vi "Log Alarm FGV.vi"(8 "error in (no error)":errorcluster, 9 "Alarm":T1, 10 "Path":path, 11 "Operation":T2) -> (0 "error out":errorcluster)   [LabVIEW 2021, in "Dynamic Shared Variables.lvlib"]
doc: "Creates, writes and closes a CSV file that contains information on alarm transitions (i.e. active, ack, cleared)."
uses:
  Dynamic Shared Variables.lvlib
  Alarm Log Operation Enum.ctl
  Tag VIs/Tag FGV Operation Enum.ctl
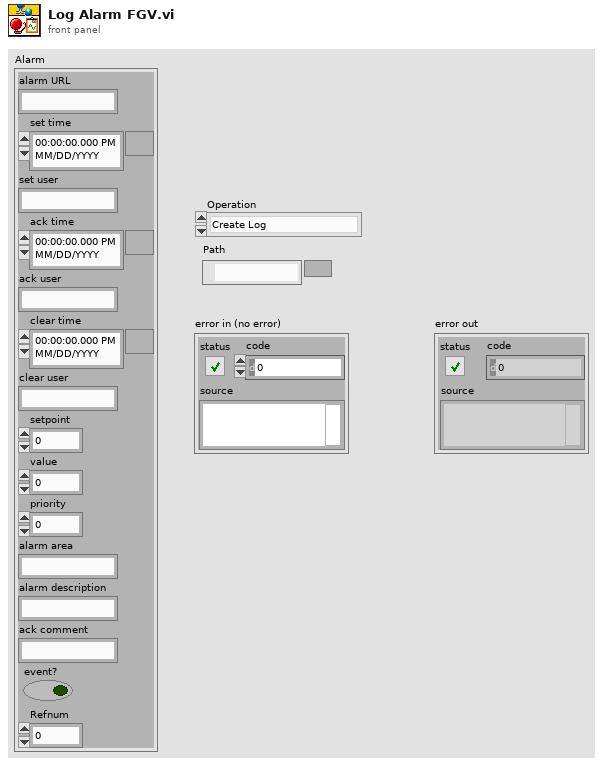
[diagram p1: front panel]
types:
  T1 = cluster{"alarm URL":string, "set time":timestamp, "set user":string, "ack time":timestamp, "ack user":string, "clear time":timestamp, "clear user":string, "setpoint":dbl, "value":dbl, "priority":u32, "alarm area":string, "alarm description":string, "ack comment":string, "event?":bool, "Refnum":u64}
  T2 = typedef "Alarm Log Operation Enum.ctl" = enum16{"Create Log", "Log Alarm", "Close Log"}
  T3 = enum16{"open", "replace", "create", "open or create", "replace or create", "replace or create with confirmation"}
  T4 = typedef "Tag FGV Operation Enum.ctl" = enum16{"Init", "Set Notification Queue", "Create Tag", "Commit", "Write Tag (Numeric)", "Write Tag (Boolean)", "Read All Tags", "Read One Tag", "Delete Tag Category", "Set Alarm Parameters (Numeric)", "Set Alarm Parameters (Boolean)", "Enable All Alarms", "Disable All Alarms", "Delete All Tags", "Read Alarms", "Ack Alarm", "Read Alarm Parameters (Numeric)", "Read Alarm Parameters (Boolean)"}
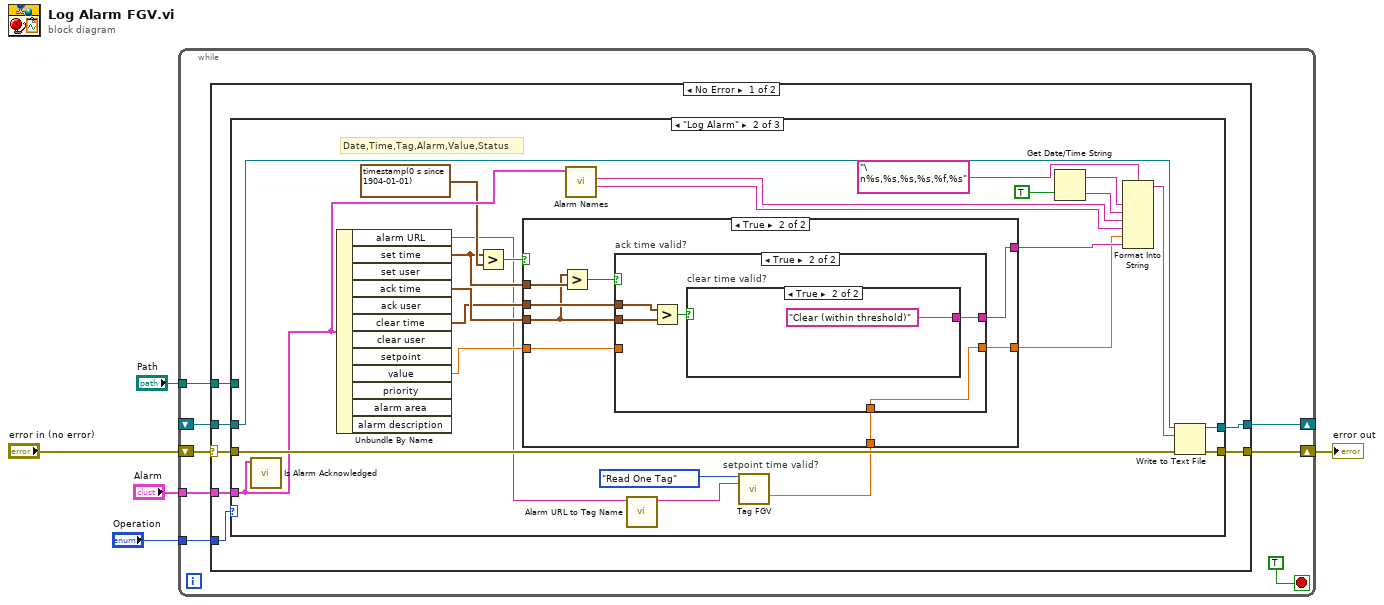
[diagram p0: block diagram]
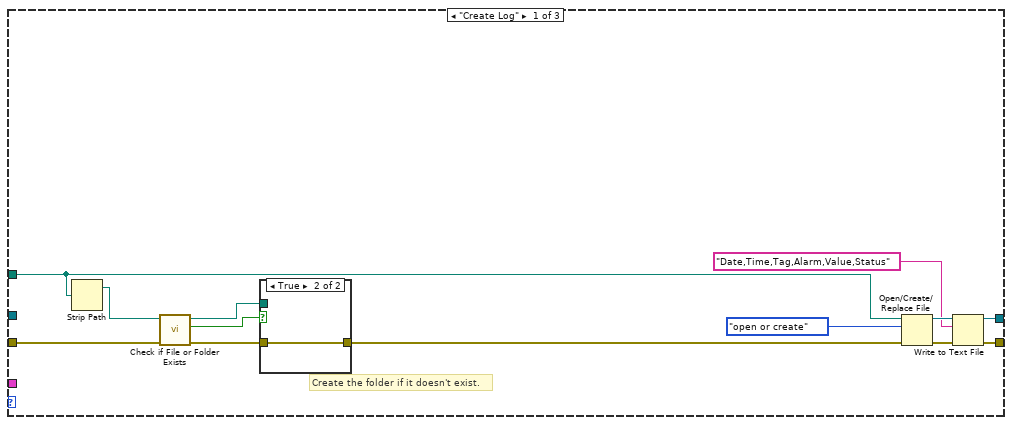
[diagram p2: hidden frame]
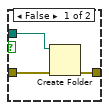
[diagram p3: hidden frame]
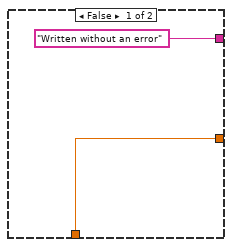
[diagram p4: hidden frame]
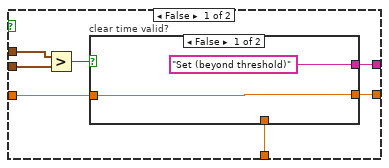
[diagram p5: hidden frame]
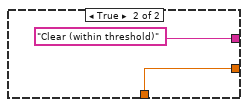
[diagram p6: hidden frame]
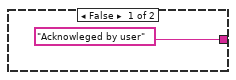
[diagram p7: hidden frame]
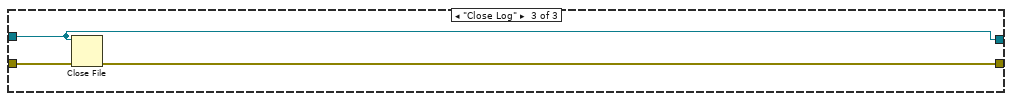
[diagram p8: hidden frame]
diagram:
  n1 = while {
    tunnel: "Operation" -> [w12]
    tunnel: "Path" -> [w11]
    shift-right: [w10] -> w4
    shift-left: "error in (no error)" -> [w13]
    tunnel: "Alarm" -> [w9]
    shift-right: [w8] -> _
    shift-left: _ -> [w7]
    stop <- TRUE stop-if-true
    n2 = case shown="No Error" w13 {
      selector: w13 -> [w18 w94]
      tunnel: w12 -> [w20 _]
      tunnel: w11 -> [w19 _]
      tunnel: [w17 w94] -> w10
      tunnel: w9 -> [w16 _]
      tunnel: [w15 w93] -> w8
      tunnel: w7 -> [w14 w93]
      frame No Error {
        n3 = case shown="\"Log Alarm\"" w20 {
          tunnel: w19 -> [w27 _ _]
          tunnel: w18 -> [w32 w58 w91]
          tunnel: [w24 w59 w90] -> w17
          tunnel: w16 -> [_ w51 _]
          tunnel: [w22 w60 w92] -> w15
          tunnel: w14 -> [_ w61 w92]
          frame "Create Log" {
            # "Create the folder if it doesn't exist."
            n4 = Strip Path(path=w27) -> (stripped path=w33:path)  [unwired: 1 out]
            n5 = call <vilib>:"Check if File or Folder Exists.vi"("error in (no error)"=w32, "path"=w33) -> ("error out"=w29:errorcluster, "file or folder exists?"=w31:bool, "dup path"=w30:path)  [unwired: 7 in]
            n6 = case shown="True" w31 {
              tunnel: w30 -> [w36 _]
              tunnel: w29 -> [w35 w37]
              tunnel: [w34 w37] -> w28
              frame False {
                n7 = Create Folder(path (use dialog)=w36, error in=w35) -> (error out=w34:errorcluster)  [unwired: 1 in, 2 out]
              }
              frame True {
              }
            }
            n8 = Open/Create/Replace File(file path (use dialog)=w27, error in=w28, operation (0:open)=T3."open or create") -> (refnum out=w23:refnum<file>, error out=w25:errorcluster)  [unwired: 3 in, 1 out]
            n9 = Write to Text File(file (use dialog)=w23, text="Date,Time,Tag,Alarm,Value,Status", error in=w25) -> (refnum out=w22:refnum<file>, error out=w24:errorcluster)  [unwired: 1 in, 1 out]
          }
          frame "Log Alarm" {
            # "Date,Time,Tag,Alarm,Value,Status"
            n10 = call "Is Alarm Acknowledged.vi"("Alarm"=w51) -> ()  [unwired: 8 in, 3 out]
            n11 = Unbundle By Name(w51) -> ("alarm URL"=w42:string, "set time"=w45:timestamp, "ack time"=w47:timestamp, "clear time"=w46:timestamp, "value"=w44:dbl)  [unwired: 7 out]
            n12 = Greater?(x=w45, y=timestamp(0 s since 1904-01-01)) -> (0:w48:bool)
            n13 = call "Alarm Names.vi"("Alarm"=w51) -> ("Alarm Name"=w53:string, "Base Tag Name"=w54:string)  [unwired: 8 in, 1 out]
            n14 = call "Alarm URL to Tag Name.vi"("alarm URL"=w42) -> ("tag name"=w39:string)  [unwired: 10 in]
            n15 = call "Tag FGV.vi"("Operation"=Tag_FGV_Operation_Enum."Read One Tag", "Tag Name"=w39) -> ("Tag Value"=w38:dbl)  [unwired: 6 in, 7 out]
            n16 = case "setpoint time valid?" shown="True" w48 {
              tunnel: ["Written without an error" w71] -> w50
              tunnel: w47 -> [_ w67]
              tunnel: w46 -> [_ w68]
              tunnel: w45 -> [_ w69]
              tunnel: [w62 w66] -> w43
              tunnel: w44 -> [_ w65]
              tunnel: w38 -> [w62 w64]
              frame False {
              }
              frame True {
                n17 = Greater?(x=w67, y=w69) -> (0:w70:bool)
                n18 = case "ack time valid?" shown="True" w70 {
                  tunnel: [w78 w87] -> w71
                  tunnel: w68 -> [w76 w85]
                  tunnel: w67 -> [w75 w84]
                  tunnel: [w74 w83] -> w66
                  tunnel: w65 -> [w73 _]
                  tunnel: w64 -> [w72 w83]
                  frame False {
                    n19 = Greater?(x=w76, y=w75) -> (0:w77:bool)
                    n20 = case "clear time valid?" shown="False" w77 {
                      tunnel: ["Set (beyond threshold)" "Clear (within threshold)"] -> w78
                      tunnel: [w79 w82] -> w74
                      tunnel: w73 -> [w79 _]
                      tunnel: w72 -> [_ w82]
                      frame False {
                      }
                      frame True {
                      }
                    }
                  }
                  frame True {
                    n21 = Greater?(x=w85, y=w84) -> (0:w86:bool)
                    n22 = case "clear time valid?" shown="True" w86 {
                      tunnel: ["Acknowleged by user" "Clear (within threshold)"] -> w87
                      frame False {
                      }
                      frame True {
                      }
                    }
                  }
                }
              }
            }
            n23 = Get Date/Time String(want seconds? (F)=TRUE) -> (date string=w56:string, time string=w55:string)  [unwired: 2 in]
            n24 = Format Into String(format string="\n%s,%s,%s,%s,%f,%s", w56, w55, w54, w53, w43, w50) -> (resulting string=w52:string)  [unwired: 2 in, 1 out]
            n25 = Write to Text File(file (use dialog)=w61, text=w52, error in=w58) -> (refnum out=w60:refnum<file>, error out=w59:errorcluster)  [unwired: 1 in, 1 out]
          }
          frame "Close Log" {
            n26 = Close File(refnum=w92, error in=w91) -> (error out=w90:errorcluster)  [unwired: 1 out]
          }
        }
      }
      frame Error {
      }
    }
  }
  "error out" <- w4
